vi "NiFPGA Download.vi"(8 "error in (no error)":errorcluster, 11 "Session":u32) -> (0 "error out":errorcluster, 3 "Session Out":u32)   [LabVIEW 2010, in "FPGA Interface Wrapper.lvlib"]
doc: "Re-downloads the FPGA bitstream to the target."
uses:
  <userlib>/_FPGA Interface Advanced Tools/FPGA Interface Wrapper/FPGA Interface Wrapper.lvlib
  NiFpga.dll
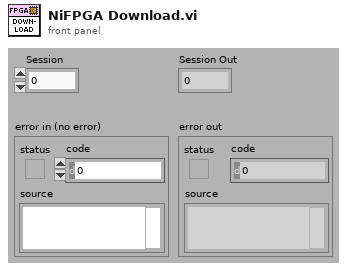
[diagram p1: front panel]
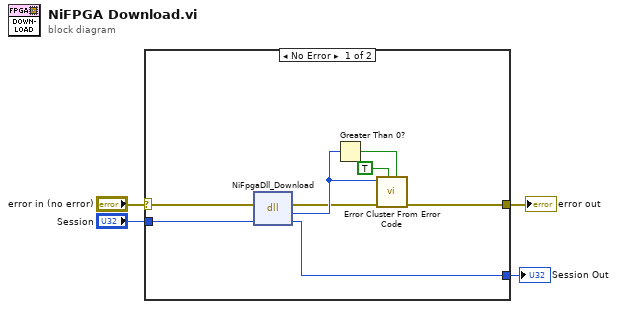
[diagram p0: block diagram]
diagram:
  n1 = case shown="No Error" "error in (no error)" {
    selector: "error in (no error)" -> [w12 w13]
    tunnel: [w5 w13] -> w3
    tunnel: "Session" -> [w11 w14]
    tunnel: [w10 w14] -> w1
    frame No Error {
      n2 = dll-call lib="NiFpga.dll" fn="NiFpgaDll_Download"(error in=w12, "Session"=w11) -> (error out=w6:errorcluster, "Status"=w7:i32, "Session"=w10:u32)  [unwired: 2 in, 1 out]
      n3 = Greater Than 0?(x=w7) -> (x > 0?=w8:bool)
      n4 = call <vilib>:"Error Cluster From Error Code.vi"("is warning? (False)"=w8, "show call chain? (False)"=TRUE, "error in (no error)"=w6, "error code (0)"=w7) -> ("error out"=w5:errorcluster)  [unwired: 5 in]
    }
    frame Error {
    }
  }
  "error out" <- w3
  "Session Out" <- w1
